vi "Pulse_Reset.vi"(2 "error in":errorcluster, 3 "reset?":bool=TRUE, 4 "VISA arduino in":refnum<visa-resource-name>) -> (0 "error out":errorcluster, 1 "VISA arduino out":refnum<visa-resource-name>)   [LabVIEW 2021]
uses:
  <vilib>/Utility/error.llb/Error Cluster From Error Code.vi
  <vilib>/ErrorRing/Error Ring.xnode
panel:
  out "delay":u32
  # "Private"
  # "Public"
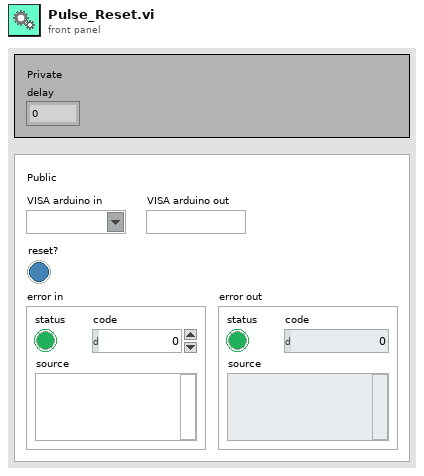
[diagram p1: front panel]
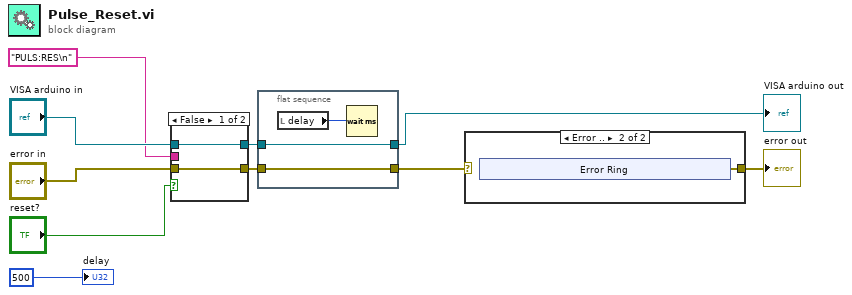
[diagram p0: block diagram]
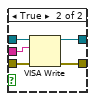
[diagram p2: hidden frame]
diagram:
  n1 = case shown="False" "reset?" {
    tunnel: [w12 w17] -> w8
    tunnel: [w11 w16] -> w7
    tunnel: "VISA arduino in" -> [w12 w15]
    tunnel: "error in" -> [w11 w14]
    tunnel: "PULS:RES\n" -> [_ w13]
    frame False {
    }
    frame True {
      n2 = VISA Write(VISA resource name=w15, write buffer=w13, error in (no error)=w14) -> (VISA resource name out=w17:refnum<visa-resource-name>, error out=w16:errorcluster)  [unwired: 1 out]
    }
  }
  n3 = flat-sequence {
    tunnel: [w20] -> w5
    tunnel: w8 -> [w20]
    tunnel: [w19] -> w9
    tunnel: w7 -> [w19]
    frame #0 {
      n4 = local read "delay"() -> (w18:u32)
      n5 = Wait (ms)(milliseconds to wait=w18) -> ()  [unwired: 1 out]
    }
  }
  n6 = case shown="Error .." w9 {
    selector: w9 -> [w21 _]
    tunnel: [w21 w22] -> w6
    frame No Error {
    }
    frame Error {
      n7 = xnode "Error Ring"() -> ("error out"=w22:errorcluster)
    }
  }
  "error out" <- w6
  "delay" <- u32 500
  "VISA arduino out" <- w5
